vi "ZL300.vi"(9 "Stage Action":T1={"Action"=enum."Get Position", "Axis"=[], "Setpoint"=[], "Velocity"=0.5, "Cmd Recvd?"=FALSE, "Position"=[], "Status"=enum."Error", "Misc"=variant} {"Velocity" min=0.0 max=1.0 step=0.01}, 10 "Stage Status":refnum<notifier>, 11 "MCL Handle":i32) -> (3 "handle out":i32)   [LabVIEW 2016]
uses:
  Stages Controls/Stage Notifier Element.ctl
  Stages Controls/Stage Actions.ctl
  Stages Controls/Stage Status.ctl
  MCL Libraries/Madlib.dll
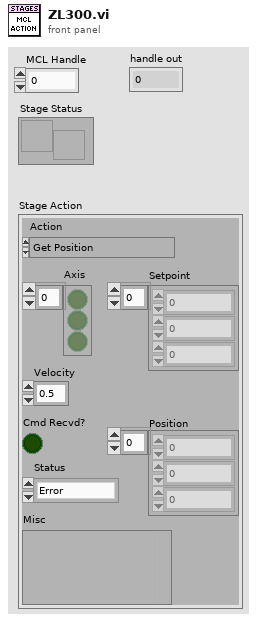
[diagram p1: front panel]
types:
  T1 = typedef "Stage Notifier Element.ctl" = cluster{"Action":T2, "Axis":bool[], "Setpoint":dbl[], "Velocity":dbl, "Cmd Recvd?":bool, "Position":dbl[], "Status":T3, "Misc":variant}
  T2 = typedef "Stage Actions.ctl" = enum16{"Get Position", "MVR", "MOVE", "HALT", "ONTARGET", "ERROR", "REFERENCE", "INIT", "VELOCITY", "STATUS", "EXIT", "HOME", "ZEROPOS", "NANOPOS", "ANALOG", "QUIT"}
  T3 = typedef "Stage Status.ctl" = enum16{"Error", "Abort", "Busy", "On Target"}
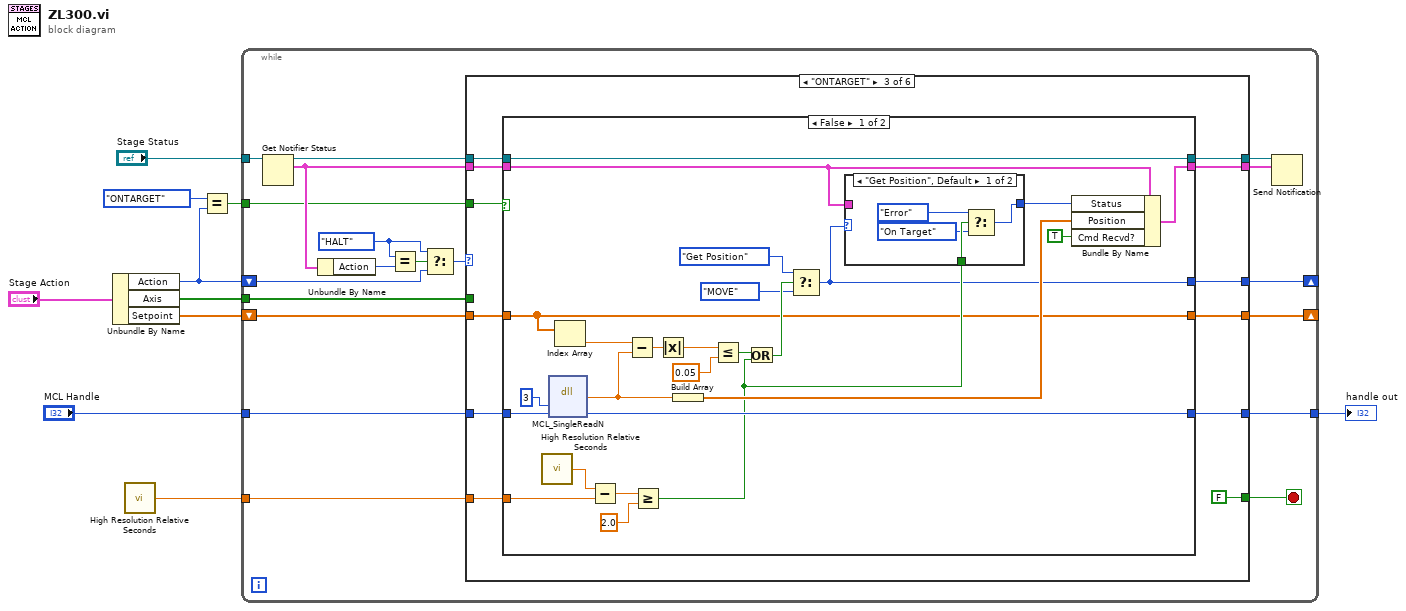
[diagram p0: block diagram]
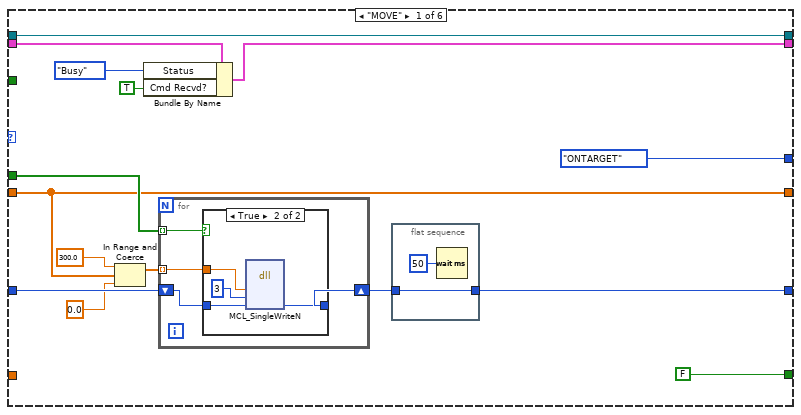
[diagram p2: hidden frame]
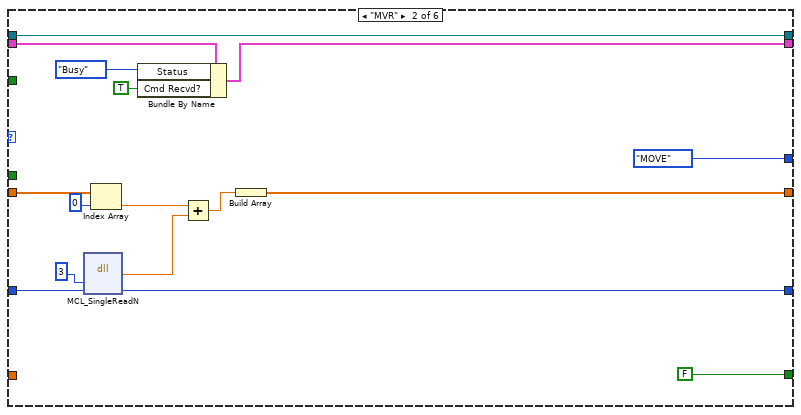
[diagram p4: hidden frame]
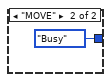
[diagram p5: hidden frame]
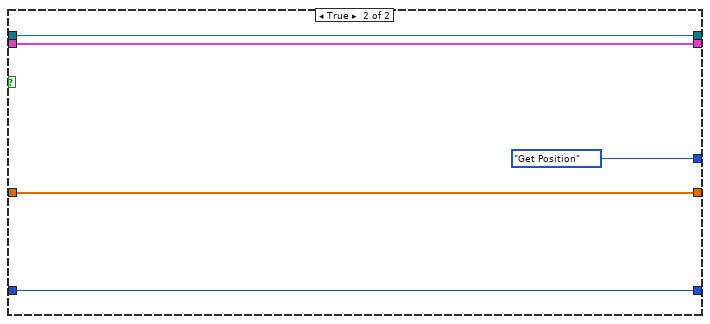
[diagram p6: hidden frame]
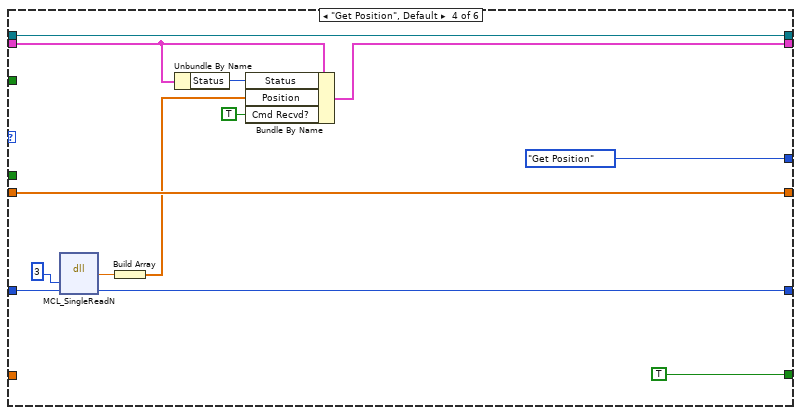
[diagram p7: hidden frame]
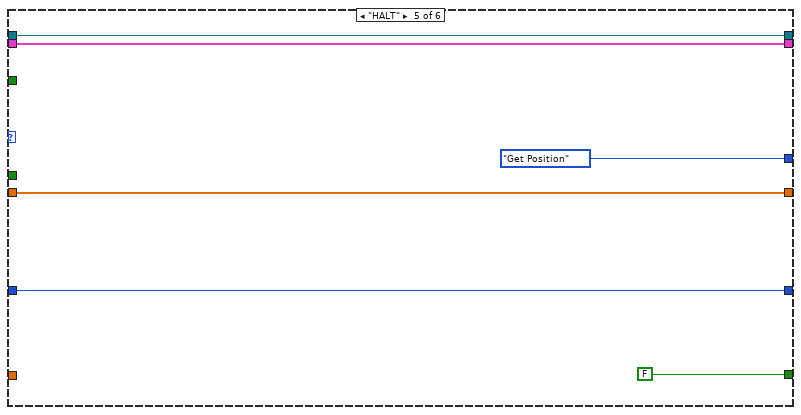
[diagram p8: hidden frame]
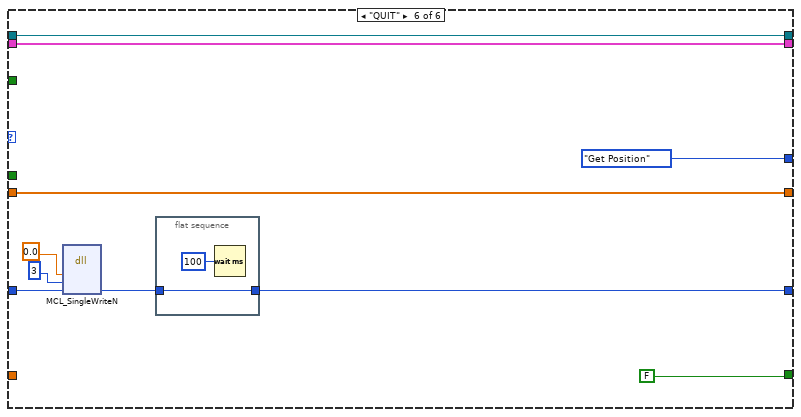
[diagram p9: hidden frame]
diagram:
  n1 = Unbundle By Name("Stage Action") -> ("Action"=w3:T2, "Axis"=w7:bool[], "Setpoint"=w6:dbl[])
  n2 = call <vilib>:"High Resolution Relative Seconds.vi"() -> ("relative seconds"=w5:dbl)
  n3 = Equal?(x=Stage_Actions."ONTARGET", y=w3) -> (x = y?=w2:bool)
  n4 = while {
    shift-right: [w27] -> _
    shift-left: w3 -> [w14]
    tunnel: "MCL Handle" -> [w28]
    tunnel: [w26] -> w10
    tunnel: w7 -> [w25]
    shift-right: [w23] -> _
    shift-left: w6 -> [w24]
    tunnel: "Stage Status" -> [w20]
    tunnel: w5 -> [w18]
    tunnel: w2 -> [w12]
    stop <- w29 stop-if-true
    w11 = Stage_Actions."HALT" ("x")
    n5 = Get Notifier Status(notifier=w20) -> (notifier out=w19:refnum<notifier>, current notification=w16:T1)  [unwired: 1 in, 3 out]
    n6 = Unbundle By Name(w16) -> ("Action"=w17:T2)
    n7 = Equal?(x=w11, y=w17) -> (x = y?=w15:bool)
    n8 = Select(t=w11, s=w15, f=w14) -> (s? t:f=w13:T2)
    n9 = case shown="\"ONTARGET\"" w13 {
      tunnel: [FALSE FALSE FALSE TRUE FALSE FALSE] -> w29
      tunnel: w28 -> [w44 w71 w83 w131 w136 w147]
      tunnel: [Stage_Actions."ONTARGET" ("x") Stage_Actions."MOVE" ("x") w76 Stage_Actions."Get Position" ("x") Stage_Actions."Get Position" ("x") Stage_Actions."Get Position" ("x")] -> w27
      tunnel: [w39 w70 w82 w130 w136 w146] -> w26
      tunnel: w25 -> [w43 _ _ _ _ _]
      tunnel: w24 -> [w41 w68 w81 w127 w137 w141]
      tunnel: [w41 w63 w73 w127 w137 w141] -> w23
      tunnel: w19 -> [w34 w59 w75 w123 w134 w140]
      tunnel: [w34 w59 w74 w123 w134 w140] -> w22
      tunnel: [w35 w61 w79 w124 w133 w139] -> w21
      tunnel: w16 -> [w33 w58 w77 w122 w133 w139]
      tunnel: w18 -> [_ _ w78 _ _ _]
      tunnel: w12 -> [_ _ w72 _ _ _]
      frame "MOVE" {
        n10 = In Range and Coerce(upper limit=300.0, x=w41, lower limit=0.0) -> (coerced(x)=w40:dbl[])  [unwired: 1 out]
        n11 = Bundle By Name(cluster=w33, "Status"=Stage_Status."Busy", "Cmd Recvd?"=TRUE) -> (w35:T1)
        n12 = for {
          shift-right: [w49] -> w38
          shift-left: w44 -> [w50]
          tunnel: w43 -> [w48] mode=indexing
          tunnel: w40 -> [w47] mode=indexing
          n13 = case shown="True" w48 {
            tunnel: w50 -> [w51 w55]
            tunnel: [w51 w54] -> w49
            tunnel: w47 -> [_ w53]
            frame False {
            }
            frame True {
              n14 = dll-call lib="C:/Users/4PiSMS/Documents/Microscope-Control/Device Library/Stages/Mad City Labs/ZL300/MCL Libraries/MADLib.dll" fn="MCL_SingleWriteN"("position"=w53, "axis"=u32 3, "handle"=w55) -> ("handle"=w54:i32)  [unwired: 6 in, 2 out]
            }
          }
        }
        n15 = flat-sequence {
          tunnel: [w46] -> w39
          tunnel: w38 -> [w46]
          frame #0 {
            n16 = Wait (ms)(milliseconds to wait=u32 50) -> ()  [unwired: 1 out]
          }
        }
      }
      frame "MVR" {
        n17 = dll-call lib="C:/Users/4PiSMS/Documents/Microscope-Control/Device Library/Stages/Mad City Labs/ZL300/MCL Libraries/MADLib.dll" fn="MCL_SingleReadN"("axis"=u32 3, "handle"=w71) -> ("return type"=w65:dbl, "handle"=w70:i32)  [unwired: 4 in, 2 out]
        n18 = Index Array(array=w68, index=0) -> (element=w66:dbl)
        n19 = Bundle By Name(cluster=w58, "Status"=Stage_Status."Busy", "Cmd Recvd?"=TRUE) -> (w61:T1)
        n20 = Add(x=w66, y=w65) -> (x+y=w64:dbl)
        n21 = Build Array(w64) -> (w63:dbl[])
      }
      frame "ONTARGET" {
        n22 = case shown="False" w72 {
          tunnel: w83 -> [w108 w115]
          tunnel: [w107 w115] -> w82
          tunnel: w81 -> [w87 w116]
          tunnel: [w97 w117] -> w79
          tunnel: w78 -> [w94 _]
          tunnel: w77 -> [w90 w117]
          tunnel: [w89 Stage_Actions."Get Position" ("x")] -> w76
          tunnel: w75 -> [w88 w118]
          tunnel: [w88 w118] -> w74
          tunnel: [w87 w116] -> w73
          frame False {
            n23 = call <vilib>:"High Resolution Relative Seconds.vi"() -> ("relative seconds"=w95:dbl)
            n24 = dll-call lib="C:/Users/4PiSMS/Documents/Microscope-Control/Device Library/Stages/Mad City Labs/ZL300/MCL Libraries/MADLib.dll" fn="MCL_SingleReadN"("axis"=u32 3, "handle"=w108) -> ("return type"=w100:dbl, "handle"=w107:i32)  [unwired: 4 in, 2 out]
            n25 = Index Array(array=w87) -> (element=w105:dbl)  [unwired: 1 in]
            n26 = Subtract(x=w95, y=w94) -> (x-y=w93:dbl)
            n27 = Subtract(x=w105, y=w100) -> (x-y=w104:dbl)
            n28 = Greater Or Equal?(x=w93, y=2.0) -> (x >= y?=w91:bool)
            n29 = Absolute Value(x=w104) -> (abs(x)=w103:dbl)
            n30 = Build Array(w100) -> (w98:dbl[])
            n31 = Less Or Equal?(x=w103, y=0.05) -> (x <= y?=w101:bool)
            n32 = Or(x=w101, y=w91) -> (x .or. y?=w99:bool)
            n33 = Select(t=Stage_Actions."Get Position" ("x"), s=w99, f=Stage_Actions."MOVE" ("x")) -> (s? t:f=w89:T2)
            n34 = case shown="\"Get Position\", Default" w89 {
              tunnel: w90 -> [_ _]
              tunnel: [w111 Stage_Status."Busy" ("Status")] -> w84
              tunnel: w91 -> [w112 _]
              frame "Get Position", Default {
                n35 = Select(t=Stage_Status."Error" ("Status"), s=w112, f=Stage_Status."On Target" ("Status")) -> (s? t:f=w111:T3)
              }
              frame "MOVE" {
              }
            }
            n36 = Bundle By Name(cluster=w90, "Status"=w84, "Position"=w98, "Cmd Recvd?"=TRUE) -> (w97:T1)
          }
          frame True {
          }
        }
      }
      frame "Get Position", Default {
        n37 = dll-call lib="C:/Users/4PiSMS/Documents/Microscope-Control/Device Library/Stages/Mad City Labs/ZL300/MCL Libraries/MADLib.dll" fn="MCL_SingleReadN"("axis"=u32 3, "handle"=w131) -> ("return type"=w128:dbl, "handle"=w130:i32)  [unwired: 4 in, 2 out]
        n38 = Build Array(w128) -> (w120:dbl[])
        n39 = Unbundle By Name(w122) -> ("Status"=w121:T3)
        n40 = Bundle By Name(cluster=w122, "Status"=w121, "Position"=w120, "Cmd Recvd?"=TRUE) -> (w124:T1)
      }
      frame "HALT" {
      }
      frame "QUIT" {
        n41 = dll-call lib="C:/Users/4PiSMS/Documents/Microscope-Control/Device Library/Stages/Mad City Labs/ZL300/MCL Libraries/MADLib.dll" fn="MCL_SingleWriteN"("position"=0.0, "axis"=u32 3, "handle"=w147) -> ("handle"=w145:i32)  [unwired: 6 in, 2 out]
        n42 = flat-sequence {
          tunnel: [w149] -> w146
          tunnel: w145 -> [w149]
          frame #0 {
            n43 = Wait (ms)(milliseconds to wait=u32 100) -> ()  [unwired: 1 out]
          }
        }
      }
    }
    n44 = Send Notification(notification=w21, notifier=w22) -> ()  [unwired: 1 in, 2 out]
  }
  "handle out" <- w10
